vi "Write to RDMA Buffer.vi"(6 "rdma session":refnum<k21>, 8 "error in":errorcluster, 9 "timeout ms (25000)":i32=25000 format="%d ms", 10 "data":u8[](array[numeric]), 11 "RDMA Transceiver in":refnum<class "RDMA Transceiver.lvclass">) -> (0 "error out":errorcluster, 1 "timed out?":bool, 3 "RDMA Transceiver out":refnum<class "RDMA Transceiver.lvclass">)   [LabVIEW 2020, in "RDMA.lvlib" / "RDMA Transceiver.lvclass"]
doc: "Writes data to RDMA buffer."
uses:
  RDMA Transceiver.lvclass
  <vilib>/rdma/rdma.llb/RDMA Acquire Send Buffer U8.vi
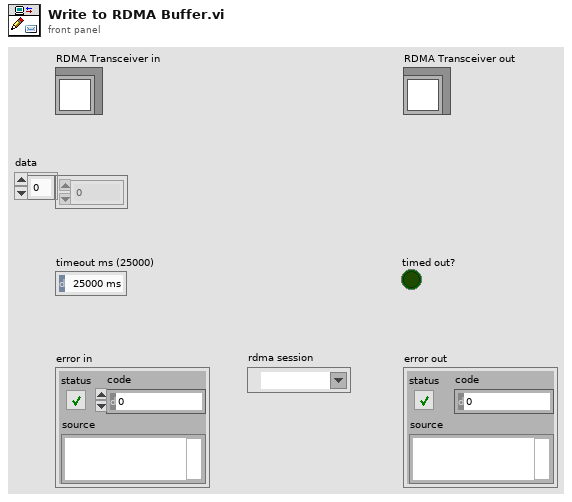
[diagram p1: front panel]
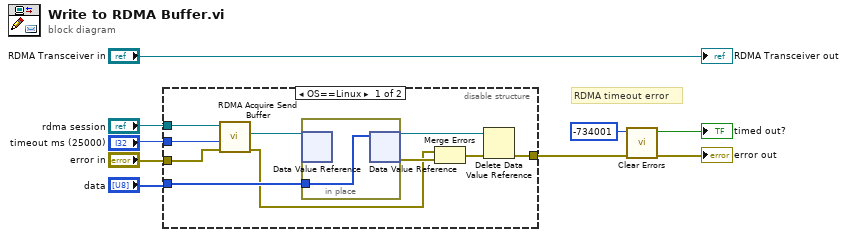
[diagram p0: block diagram]
diagram:
  # "RDMA timeout error"
  n1 = disable-structure shown="OS==Linux" {
    disable-tunnel: "data" -> [w12 _]
    disable-tunnel: "rdma session" -> [w11 _]
    disable-tunnel: "timeout ms (25000)" -> [w19 _]
    disable-tunnel: "error in" -> [w15 _]
    disable-tunnel: [w13 _] -> w4
    frame condition #0 (active) {
      n2 = call-poly <vilib>:"RDMA Acquire Send Buffer.vi"("error in"=w15, "timeout (ms)"=w19, "rdma session in"=w11) -> ("error out"=w10:errorcluster, "edvr"=w18:refnum<data-value>)  [unwired: 6 in, 1 out]
      n3 = in-place {
        in-place-border: w12 -> [w20]
        n4 = in-place-dvr #1(w18) -> ()  [unwired: 2 out]
        n5 = in-place-dvr #1(w20) -> (w16:refnum<data-value>, w17:errorcluster)
      }
      n6 = Merge Errors(w10, w17) -> (w14:errorcluster)
      n7 = Delete Data Value Reference(data value reference=w16, error in=w14) -> (error out=w13:errorcluster)  [unwired: 1 out]
    }
    frame condition #1 {
    }
  }
  n8 = call <vilib>:"Clear Errors.vi"("error in (no error)"=w4, "specific error code to clear (0: all)"=-734001) -> ("error out"=→"error out":errorcluster, "specific error cleared?"=→"timed out?":bool)  [unwired: 4 in]
  "RDMA Transceiver out" <- "RDMA Transceiver in"
